vi "Parse-device-identifier.vi"(8 "error in (no error)":errorcluster, 10 "Multiple device identification XML string":string="<LECList><LEC name=\"EC1000 (00:50:c2:4f:a4:b0)\" ip=\"128.178.146.163\" mac=\"00:50:c2:4f:a4:b0\" /></LECList>") -> (0 "error out":errorcluster, 2 "Device identifiers":T1[](array[typedef]))   [LabVIEW 2013, in "EC1000-control.lvlib" / "SM1000-control.lvclass"]
uses:
  SM1000-control.lvclass
  Device-identification.ctl
  <vilib>/xml/Load XML String.vi
  <vilib>/xml/Close Reference(Node).vi
  <vilib>/xml/Close Reference(NNMap).vi
  <vilib>/xml/NI_XML.lvlib
  <resource>/objmgr/DOMUserDefRef.rc
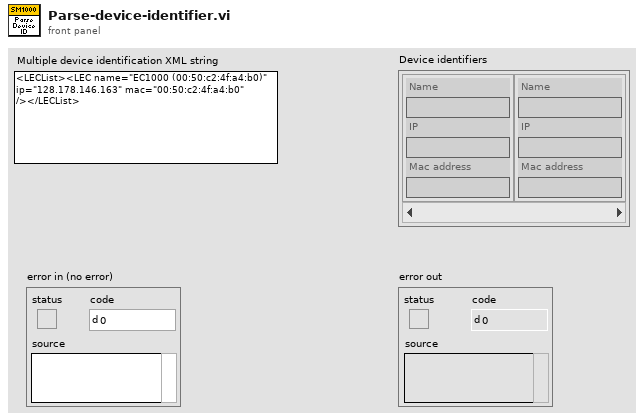
[diagram p1: front panel]
types:
  T1 = typedef "EC1000-control.lvlib/SM1000-control.lvclass/Device-identification.ctl" = cluster{"Name":string, "IP":string, "Mac address":string}
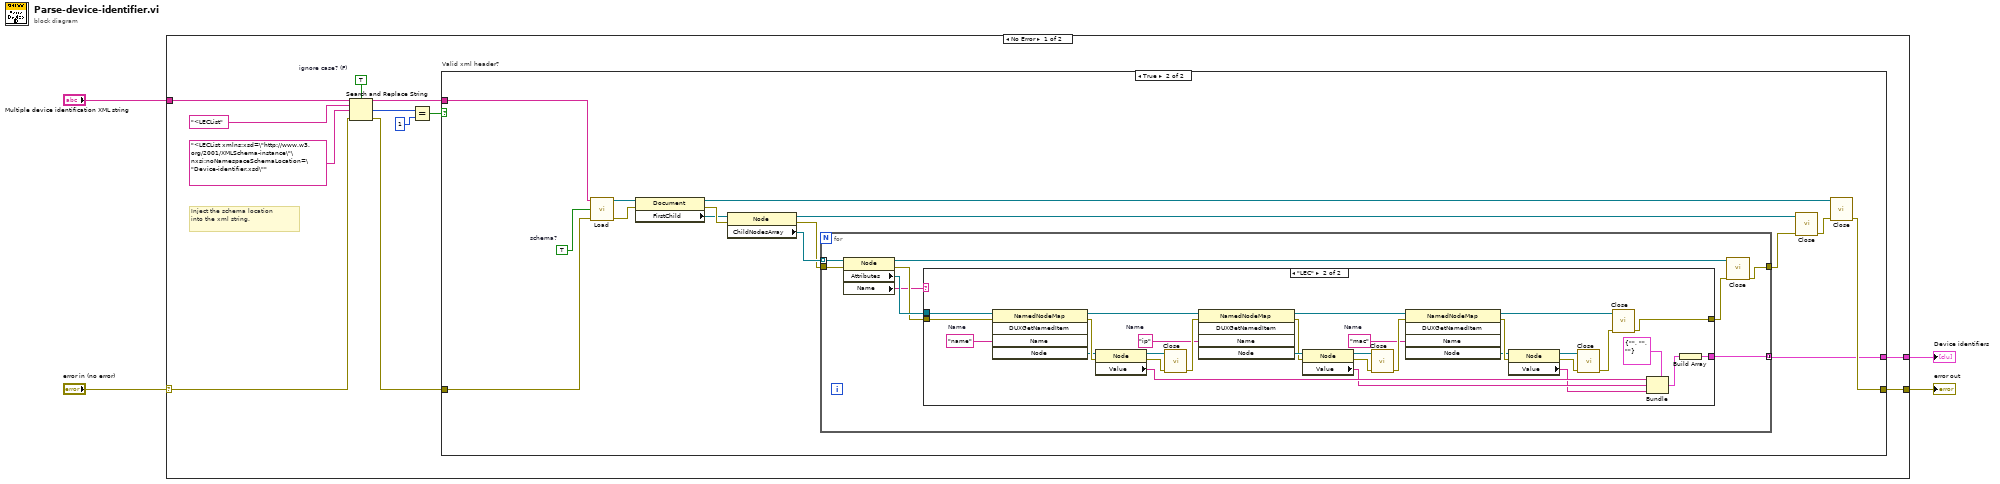
[diagram p0: block diagram]
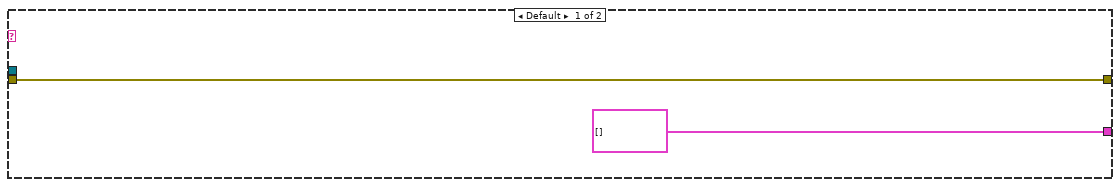
[diagram p3: hidden frame]
diagram:
  n1 = case shown="No Error" "error in (no error)" {
    selector: "error in (no error)" -> [w13 w74]
    tunnel: [w8 w74] -> w3
    tunnel: "Multiple device identification XML string" -> [w16 _]
    tunnel: [w6 _] -> w1
    frame No Error {
      w5 = TRUE  # ignore case? (F)
      # "Inject the schema location\ninto the xml string."
      n2 = Search and Replace String(case sensitive?=w5, input string=w16, search string="<LECList", replace string="<LECList xmlns:xsd=\"http://www.w3.org/2001/XMLSchema-instance\"\nxsi:noNamespaceSchemaLocation=\"Device-identifier.xsd\"", error in=w13) -> (result string=w9:string, number of replacements=w12:i32, error out=w7:errorcluster)  [unwired: 3 in, 1 out]
      n3 = Equal?(x=w12, y=1) -> (x = y?=w10:bool)
      n4 = case "Valid xml header?" shown="True" w10 {
        tunnel: w9 -> [_ w18]
        tunnel: [w17 w28] -> w8
        tunnel: w7 -> [w17 w29]
        tunnel: [_ w25] -> w6
        frame False {
        }
        frame True {
          w32 = TRUE  # schema?
          n5 = call-poly <vilib>:"Load.vi"("XML string"=w18, "process schema (False)"=w32, "error in (no error)"=w29) -> ("DOM document out"=w31:refnum<k20>, "error out"=w30:errorcluster)  [unwired: 10 in, 1 out]
          n6 = property class="Document"(reference=w31, error in=w30) -> (reference out=w20:refnum<k20>, error out=w22:errorcluster, "FirstChild"=w19:refnum<k20>)
          n7 = property class="Node"(reference=w19, error in=w22) -> (reference out=w21:refnum<k20>, error out=w23:errorcluster, "ChildNodesArray"=w24:refnum<k20>[])
          n8 = for {
            tunnel: w24 -> [w41] mode=indexing
            tunnel: [w37] -> w25 mode=concatenating
            tunnel: w23 -> [w40]
            tunnel: [w34] -> w27
            n9 = property class="Node"(reference=w41, error in=w40) -> (reference out=w36:refnum<k20>, error out=w38:errorcluster, "Attributes"=w39:refnum<k20>, "Name"=w33:string)
            n10 = case shown="\"LEC\"" w33 {
              tunnel: w39 -> [_ w73]
              tunnel: w38 -> [w43 w72]
              tunnel: [T1[] [] w47] -> w37
              tunnel: [w43 w52] -> w35
              frame Default {
              }
              frame "LEC" {
                w53 = "mac"  # Name
                w60 = "ip"  # Name
                w67 = "name"  # Name
                n11 = invoke class="NamedNodeMap" method="DUXGetNamedItem"(reference=w73, error in=w72, "Name"=w67) -> (reference out=w62:refnum<k20>, error out=w71:errorcluster, "Node"=w68:refnum<k20>)  [unwired: 2 in, 2 out]
                n12 = property class="Node"(reference=w68, error in=w71) -> (reference out=w70:refnum<k20>, error out=w69:errorcluster, "Value"=w46:string)
                n13 = call-poly <vilib>:"Close.vi"("error in (no error)"=w69, "node"=w70) -> ("error out"=w61:errorcluster)  [unwired: 7 in]
                n14 = invoke class="NamedNodeMap" method="DUXGetNamedItem"(reference=w62, error in=w61, "Name"=w60) -> (reference out=w55:refnum<k20>, error out=w63:errorcluster, "Node"=w66:refnum<k20>)  [unwired: 2 in, 2 out]
                n15 = property class="Node"(reference=w66, error in=w63) -> (reference out=w64:refnum<k20>, error out=w65:errorcluster, "Value"=w45:string)
                n16 = call-poly <vilib>:"Close.vi"("error in (no error)"=w65, "node"=w64) -> ("error out"=w54:errorcluster)  [unwired: 7 in]
                n17 = invoke class="NamedNodeMap" method="DUXGetNamedItem"(reference=w55, error in=w54, "Name"=w53) -> (reference out=w51:refnum<k20>, error out=w59:errorcluster, "Node"=w56:refnum<k20>)  [unwired: 2 in, 2 out]
                n18 = property class="Node"(reference=w56, error in=w59) -> (reference out=w58:refnum<k20>, error out=w57:errorcluster, "Value"=w44:string)
                n19 = call-poly <vilib>:"Close.vi"("error in (no error)"=w57, "node"=w58) -> ("error out"=w50:errorcluster)  [unwired: 7 in]
                n20 = call-poly <vilib>:"Close.vi"("error in (no error)"=w50, "named node map"=w51) -> ("error out"=w52:errorcluster)  [unwired: 7 in]
                n21 = Bundle(cluster=T1 {"Name"="", "IP"="", "Mac address"=""} ("Device"), "Name"=w46, "IP"=w45, "Mac address"=w44) -> (w48:T1)
                n22 = Build Array(w48) -> (w47:T1[])
              }
            }
            n23 = call-poly <vilib>:"Close.vi"("error in (no error)"=w35, "node"=w36) -> ("error out"=w34:errorcluster)  [unwired: 7 in]
          }
          n24 = call-poly <vilib>:"Close.vi"("error in (no error)"=w27, "node"=w21) -> ("error out"=w26:errorcluster)  [unwired: 7 in]
          n25 = call-poly <vilib>:"Close.vi"("error in (no error)"=w26, "node"=w20) -> ("error out"=w28:errorcluster)  [unwired: 7 in]
        }
      }
    }
    frame Error {
    }
  }
  "error out" <- w3
  "Device identifiers" <- w1
